vi "EPS-Release.vi"(8 "error in":errorcluster, 11 "EPS Setting":T1) -> (0 "error out":errorcluster)   [LabVIEW 2018]
uses:
  Data Def/EPS-Setting.ctl
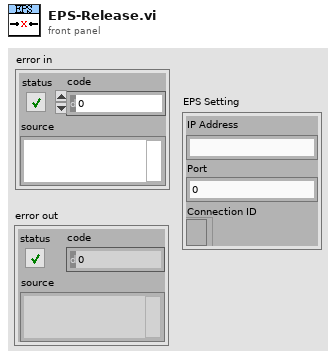
[diagram p1: front panel]
types:
  T1 = typedef "EPS-Setting.ctl" = cluster{"IP Address":string, "Port":u16, "Connection ID":refnum<k5>}
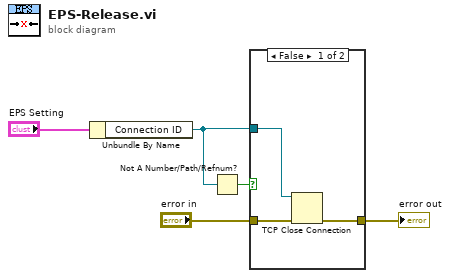
[diagram p0: block diagram]
diagram:
  n1 = Unbundle By Name("EPS Setting") -> ("Connection ID"=w1:refnum<k5>)
  n2 = Not A Number/Path/Refnum?(number/path/refnum=w1) -> (NaN/Path/Refnum?=w2:bool)
  n3 = case shown="False" w2 {
    tunnel: w1 -> [w8 _]
    tunnel: "error in" -> [w7 w9]
    tunnel: [w6 w9] -> w3
    frame False {
      n4 = TCP Close Connection(connection ID=w8, error in (no error)=w7) -> (error out=w6:errorcluster)  [unwired: 1 in, 1 out]
    }
    frame True {
    }
  }
  "error out" <- w3
